vi "SQL_users_find.vi"(11 "用户名":string) -> (2 "error out":errorcluster, 3 "是否存在该用户":bool)   [LabVIEW 2014]
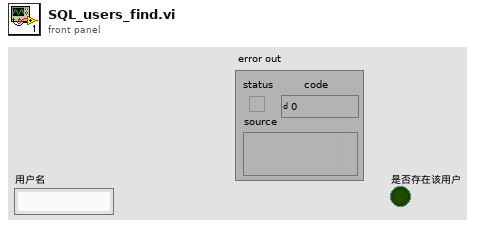
[diagram p1: front panel]
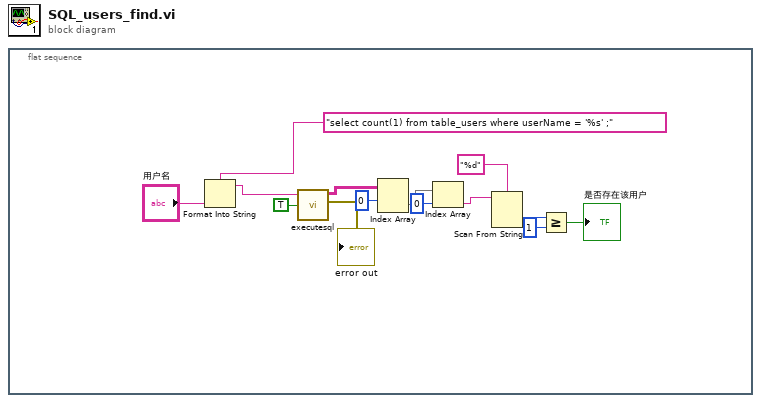
[diagram p0: block diagram]
diagram:
  n1 = flat-sequence {
    frame #0 {
      n2 = Format Into String(format string="select count(1) from table_users where userName = '%s' ;" ("Command Text"), "用户名") -> (resulting string=w13:string)  [unwired: 2 in, 1 out]
      n3 = call "executesql.vi"("Return Data (T)"=TRUE, "Command Text"=w13) -> ("error out"=→"error out":errorcluster, "Data"=w10:string[][])  [unwired: 5 in]
      n4 = Index Array(array=w10, index (row)=0 ("索引 (行)")) -> (element=w8:string[])  [unwired: 1 in]
      n5 = Index Array(array=w8, index=0 ("索引")) -> (element=w6:string)
      n6 = Scan From String(format string="%d" ("格式字符串"), input string=w6) -> (output 1=w4:i32)  [unwired: 3 in, 3 out]
      n7 = Greater Or Equal?(x=w4, y=1) -> (x >= y?=→"是否存在该用户":bool)
    }
  }
